vi "ReadStatusOk.vi"(8 "error in (no error)":errorcluster, 11 "object in":refnum<class "Reply Message.lvclass">) -> (0 "error out":errorcluster, 2 "status ok":bool, 3 "object out":refnum<class "Reply Message.lvclass">)   [LabVIEW 2018, in "ClientMessaging.lvlib" / "Reply Message.lvclass"]
uses:
  Reply Message.lvclass
  Reply Message.lvclass/Reply Message.ctl
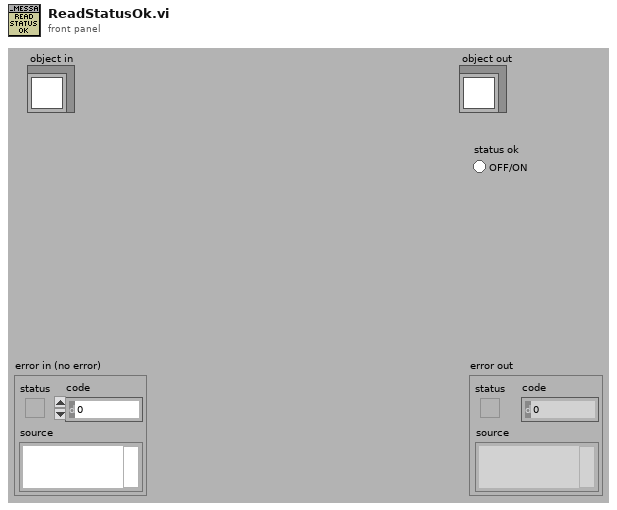
[diagram p1: front panel]
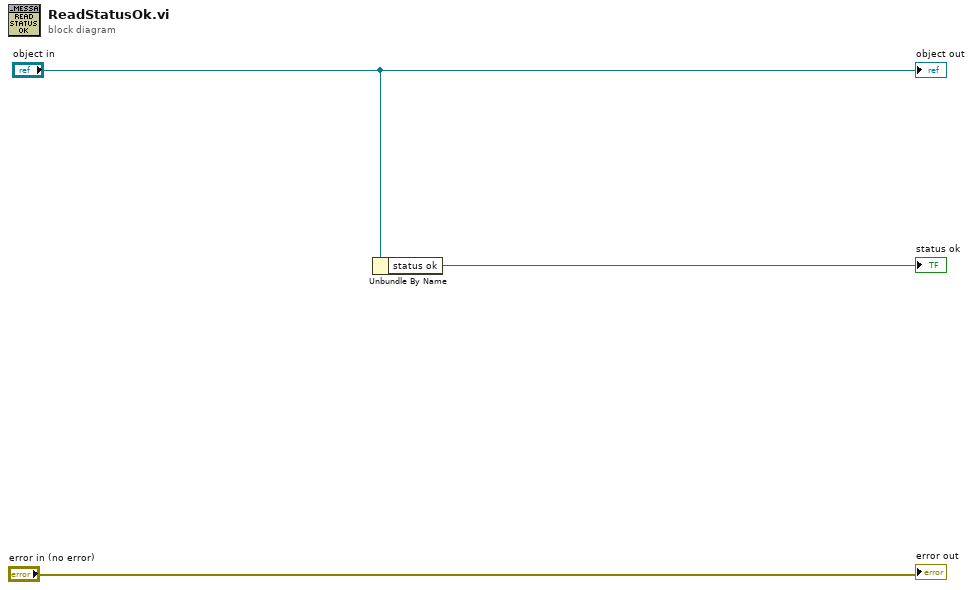
[diagram p0: block diagram]
diagram:
  n1 = Unbundle By Name("object in") -> ("status ok"=→"status ok":bool)
  "error out" <- "error in (no error)"
  "object out" <- "object in"
